vi "Configure PA UTSIGNAL query.vi"(8 "error in (no error)":errorcluster, 11 "VISA resource in":refnum<visa-resource-name>) -> (0 "error out":errorcluster, 2 "UTS":string, 3 "VISA resource out":refnum<visa-resource-name>)   [LabVIEW 2025, in "Chroma 19052.lvlib"]
uses:
  <instrlib>/Chroma 19052/Chroma 19052.lvlib
  <instrlib>/Chroma 19052/Public/Utility/Type Def/steps--numeric.ctl
panel:
  in  "Step":T1=1 min=1 max=99 step=1
  # "0 = OFF\n1 = ON"
  # "Get UT SIGNAL on/off"
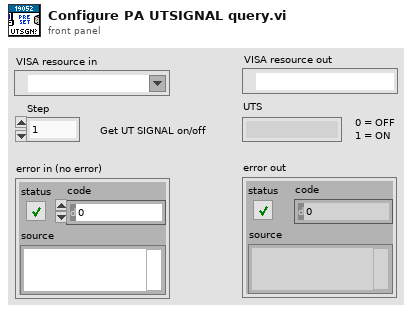
[diagram p1: front panel]
types:
  T1 = typedef "Chroma 19052.lvlib/steps--numeric.ctl" = u8
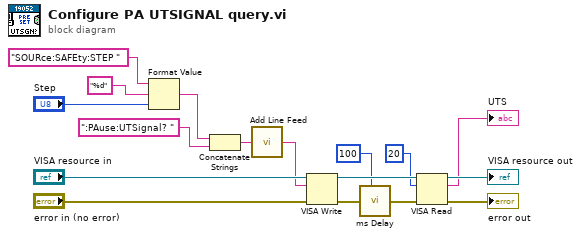
[diagram p0: block diagram]
diagram:
  n1 = Format Value(string ("")="SOURce:SAFEty:STEP ", format string="%d", value (0)="Step") -> (output string=w11:string)
  n2 = Concatenate Strings(w11, ":PAuse:UTSignal? ") -> (w4:string)
  n3 = call <instrlib>:"Add Line Feed.vi"("Command string"=w4) -> ("Concatenated string"=w3:string)  [unwired: 4 in]
  n4 = VISA Write(VISA resource name="VISA resource in", write buffer=w3, error in (no error)="error in (no error)") -> (VISA resource name out=w9:refnum<visa-resource-name>, error out=w7:errorcluster)  [unwired: 1 out]
  n5 = call <instrlib>:"ms Delay.vi"("miliseconds to wait"=u32 100, "error in (no error)"=w7) -> ("error out"=w6:errorcluster)  [unwired: 6 in, 1 out]
  n6 = VISA Read(VISA resource name=w9, byte count=u32 20, error in (no error)=w6) -> (VISA resource name out=→"VISA resource out":refnum<visa-resource-name>, read buffer=→"UTS":string, error out=→"error out":errorcluster)  [unwired: 1 out]
